vi "超标留样启动流程.vi"() -> ()   [LabVIEW 2016, in "超标留样集成.lvlib" / "科盛超标留样.lvlib"]
panel:
  in  "error in (no error)":errorcluster
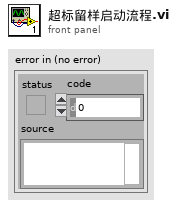
[diagram p1: front panel]
types:
  T1 = enum16{"触发采样", "触发采样完成", "供样命令", "供样完成", "留样命令", "留样完成"}
  T2 = cluster{"STEP":enum16{"open", "read", "write", "close"}, "写入缓冲区":string}
  T3 = cluster{"采样模式":enum16{"定时定量1", "定时定量2", "定流定量", "定时比例", "同步留样", "超标留样", "触发采样", "定时采样1", "定流供样", "定时采样2", "远程取样", "手动取样", "流量跟踪"}, "仪器状态":enum16{"待机", "运行中"}, "仪器时间":string, "瞬时流速(m3/s)":dbl, "当前COD值(mg/L)":dbl, "当前氨氮值(mg/L)":dbl, "当前温度(℃)":dbl, "开关量状态1":string, "开关量状态2":string, "开关量状态3":string, "A桶水样量(mL)":dbl, "B桶水样量(mL)":dbl}
  T4 = cluster{"采样泵1停0转":bool, "供样泵1停0转":bool, "泵1正转0反转":bool, "A桶搅拌1关0开":bool, "B桶搅拌1关0开":bool, "电控锁1关0开":bool, "流程1未完成0完成":bool, "外控泵1关0开":bool}
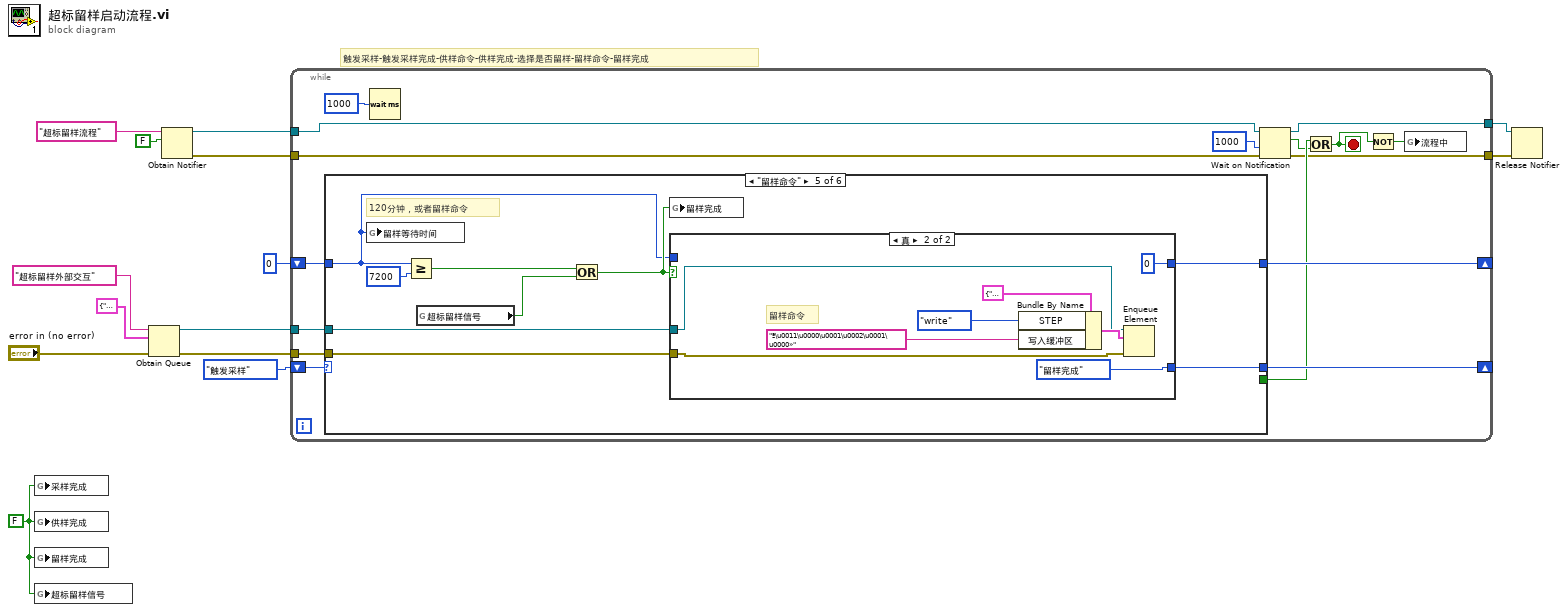
[diagram p0: block diagram]
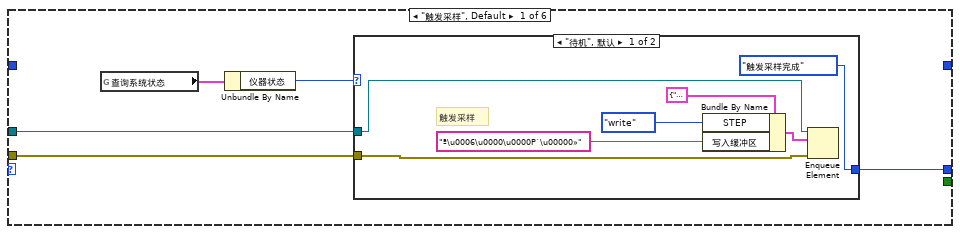
[diagram p2: hidden frame]
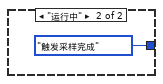
[diagram p3: hidden frame]
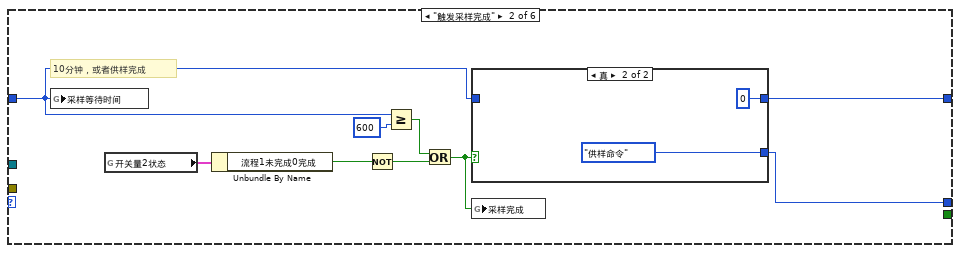
[diagram p4: hidden frame]
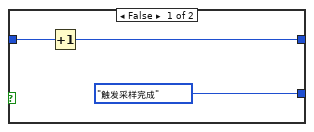
[diagram p5: hidden frame]
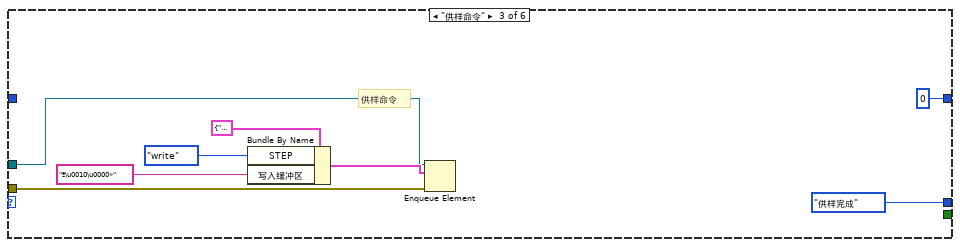
[diagram p6: hidden frame]
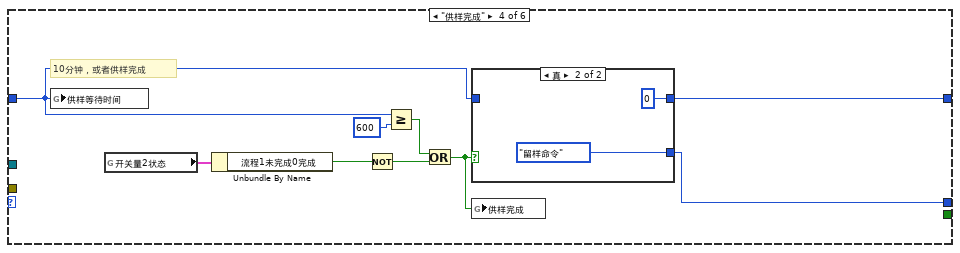
[diagram p7: hidden frame]
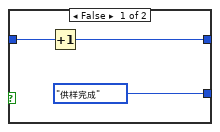
[diagram p8: hidden frame]
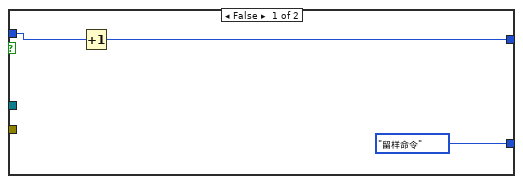
[diagram p9: hidden frame]
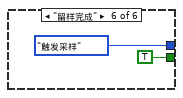
[diagram p10: hidden frame]
diagram:
  w3 = FALSE ("采样完成")
  # "触发采样-触发采样完成-供样命令-供样完成-选择是否留样-留样命令-留样完成"
  n1 = global write "超标留样全局.vi" "采样完成"(w3) -> ()
  n2 = global write "超标留样全局.vi" "供样完成"(w3) -> ()
  n3 = global write "超标留样全局.vi" "留样完成"(w3) -> ()
  n4 = global write "超标留样全局.vi" "超标留样信号"(w3) -> ()
  n5 = Obtain Queue(name (unnamed)="超标留样外部交互" ("名称（未命名）"), element data type=T2 {"STEP"=enum."write", "写入缓冲区"="ª\u0006\u0000\u0000P`\u00000»"}, error in (no error)="error in (no error)") -> (queue out=w10:refnum<queue>, error out=w9:errorcluster)  [unwired: 2 in, 1 out]
  n6 = Obtain Notifier(name (unnamed)="超标留样流程" ("名称（未命名）"), notification data type=FALSE ("采样完成")) -> (notifier out=w5:refnum<notifier>, error out=w4:errorcluster)  [unwired: 2 in, 1 out]
  n7 = while {
    shift-right: [w27] -> _
    shift-left: T1."触发采样" -> [w30]
    tunnel: w10 -> [w29]
    tunnel: w9 -> [w28]
    shift-right: [w24] -> _
    shift-left: 0 -> [w25]
    tunnel: w5 -> [w21]
    tunnel: w4 -> [w20]
    tunnel: [w16] -> w2
    tunnel: [w15] -> w1
    stop <- w18 stop-if-true
    n8 = case shown="\"留样命令\"" w30 {
      tunnel: w29 -> [w33 _ w61 _ w85 _]
      tunnel: w28 -> [w32 _ w60 _ w84 _]
      tunnel: [w31 w47 T1."供样完成" w67 w83 T1."触发采样"] -> w27
      tunnel: w25 -> [_ w44 _ w66 w80 _]
      tunnel: [_ w46 0 w68 w82 _] -> w24
      tunnel: [_ _ _ _ _ TRUE] -> w22
      frame "触发采样", Default {
        n9 = global read "超标留样全局.vi" "查询系统状态"() -> (w34:T3)
        n10 = Unbundle By Name(w34) -> ("仪器状态"=w35:enum16{"待机", "运行中"})
        n11 = case shown="\"待机\", 默认" w35 {
          tunnel: w33 -> [w38 _]
          tunnel: w32 -> [w37 _]
          tunnel: [T1."触发采样完成" T1."触发采样完成"] -> w31
          frame "待机", Default {
            # "触发采样"
            n12 = Bundle By Name(cluster=T2 {"STEP"=enum."open", "写入缓冲区"=""} ("元素"), "STEP"=enum16{"open", "read", "write", "close"}."write", "写入缓冲区"="ª\u0006\u0000\u0000P`\u00000»") -> (w41:T2)
            n13 = Enqueue Element(queue=w38, element=w41, error in (no error)=w37) -> ()  [unwired: 1 in, 3 out]
          }
          frame "运行中" {
          }
        }
      }
      frame "触发采样完成" {
        # "10分钟，或者供样完成"
        n14 = global write "超标留样全局.vi" "采样等待时间"(w44) -> ()
        n15 = global read "超标留样全局.vi" "开关量2状态"() -> (w51:T4)
        n16 = Unbundle By Name(w51) -> ("流程1未完成0完成"=w49:bool)
        n17 = Not(x=w49) -> (.not. x?=w48:bool)
        n18 = Greater Or Equal?(x=w44, y=600) -> (x >= y?=w50:bool)
        n19 = Or(x=w50, y=w48) -> (x .or. y?=w45:bool)
        n20 = case shown="真" w45 {
          tunnel: [T1."触发采样完成" T1."供样命令"] -> w47
          tunnel: w44 -> [w54 _]
          tunnel: [w53 0] -> w46
          frame False {
            n21 = Increment(x=w54) -> (x+1=w53:i32)
          }
          frame True {
          }
        }
        n22 = global write "超标留样全局.vi" "采样完成"(w45) -> ()
      }
      frame "供样命令" {
        # "供样命令"
        n23 = Bundle By Name(cluster=T2 {"STEP"=enum."open", "写入缓冲区"=""} ("元素"), "STEP"=enum16{"open", "read", "write", "close"}."write", "写入缓冲区"="ª\u0010\u0000»") -> (w64:T2)
        n24 = Enqueue Element(queue=w61, element=w64, error in (no error)=w60) -> ()  [unwired: 1 in, 3 out]
      }
      frame "供样完成" {
        # "10分钟，或者供样完成"
        n25 = global write "超标留样全局.vi" "供样等待时间"(w66) -> ()
        n26 = global read "超标留样全局.vi" "开关量2状态"() -> (w73:T4)
        n27 = Unbundle By Name(w73) -> ("流程1未完成0完成"=w71:bool)
        n28 = Not(x=w71) -> (.not. x?=w70:bool)
        n29 = Greater Or Equal?(x=w66, y=600) -> (x >= y?=w72:bool)
        n30 = Or(x=w72, y=w70) -> (x .or. y?=w69:bool)
        n31 = case shown="真" w69 {
          tunnel: [T1."供样完成" T1."留样命令"] -> w67
          tunnel: w66 -> [w76 _]
          tunnel: [w75 0] -> w68
          frame False {
            n32 = Increment(x=w76) -> (x+1=w75:i32)
          }
          frame True {
          }
        }
        n33 = global write "超标留样全局.vi" "供样完成"(w69) -> ()
      }
      frame "留样命令" {
        # "120分钟，或者留样命令"
        n34 = global write "超标留样全局.vi" "留样等待时间"(w80) -> ()
        n35 = Greater Or Equal?(x=w80, y=7200) -> (x >= y?=w87:bool)
        n36 = global read "超标留样全局.vi" "超标留样信号"() -> (w86:bool)
        n37 = Or(x=w87, y=w86) -> (x .or. y?=w81:bool)
        n38 = global write "超标留样全局.vi" "留样完成"(w81) -> ()
        n39 = case shown="真" w81 {
          tunnel: [T1."留样命令" T1."留样完成"] -> w83
          tunnel: w80 -> [w90 _]
          tunnel: [w89 0] -> w82
          tunnel: w85 -> [_ w93]
          tunnel: w84 -> [_ w92]
          frame False {
            n40 = Increment(x=w90) -> (x+1=w89:i32)
          }
          frame True {
            # "留样命令"
            n41 = Bundle By Name(cluster=T2 {"STEP"=enum."open", "写入缓冲区"=""} ("元素"), "STEP"=enum16{"open", "read", "write", "close"}."write", "写入缓冲区"="ª\u0011\u0000\u0001\u0002\u0001\u0000»") -> (w95:T2)
            n42 = Enqueue Element(queue=w93, element=w95, error in (no error)=w92) -> ()  [unwired: 1 in, 3 out]
          }
        }
      }
      frame "留样完成" {
      }
    }
    n43 = Wait (ms)(milliseconds to wait=u32 1000 ("等待时间（毫秒）")) -> ()  [unwired: 1 out]
    n44 = Wait on Notification(notifier=w21, timeout in ms (-1)=1000 ("超时毫秒(-1)"), error in (no error)=w20) -> (notifier out=w16:refnum<notifier>, notification=w17:bool, error out=w15:errorcluster)  [unwired: 1 in, 1 out]
    n45 = Or(x=w22, y=w17) -> (x .or. y?=w18:bool)
    n46 = Not(x=w18) -> (.not. x?=w23:bool)
    n47 = global write "超标留样全局.vi" "流程中"(w23) -> ()
  }
  n48 = Release Notifier(notifier=w2, error in (no error)=w1) -> ()  [unwired: 1 in, 3 out]
